vi "get_input_configuration.vi"(8 "error in (no error)":errorcluster, 11 "connection ID":refnum<k5>) -> (0 "error out":errorcluster, 1 "Sensor info 1":T1="1", 2 "Sensor type":T2="0", 3 "connection ID out":refnum<k5>, 4 "Sensor info 2":string)   [LabVIEW 2018]
uses:
  typedefs/sensor_types.ctl
  typedefs/thermocouple_types.ctl
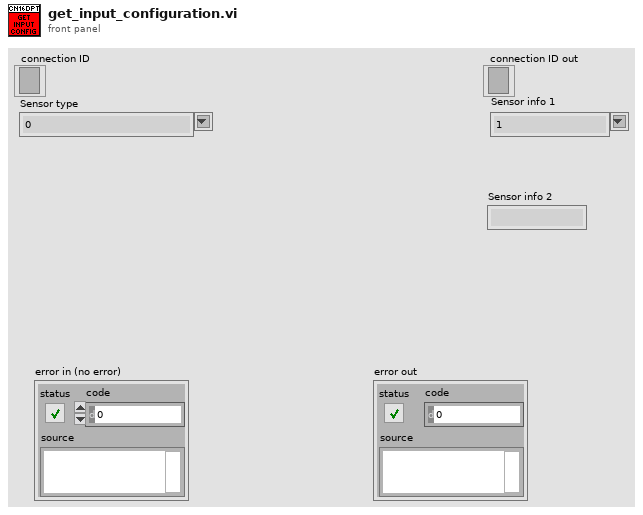
[diagram p1: front panel]
types:
  T1 = typedef "thermocouple_types.ctl" = string
  T2 = typedef "sensor_types.ctl" = string
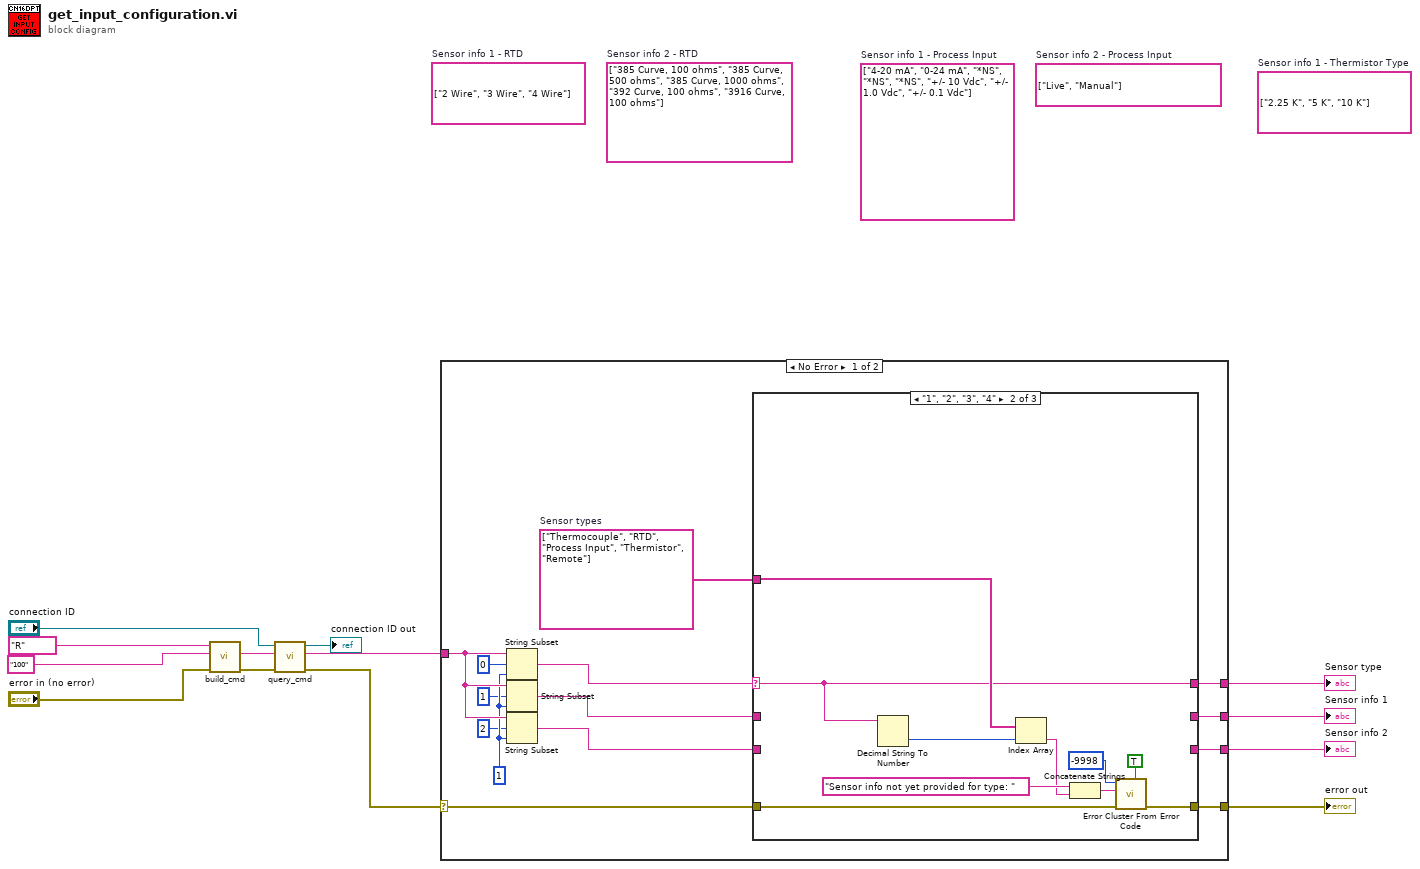
[diagram p0: block diagram]
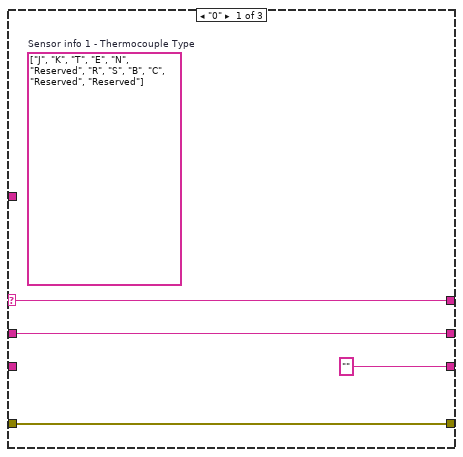
[diagram p2: hidden frame]
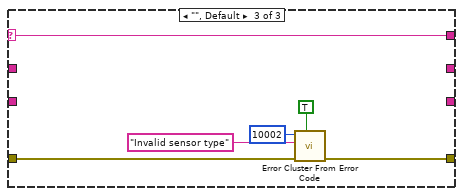
[diagram p3: hidden frame]
diagram:
  (unwired) string[] ["2.25 K", "5 K", "10 K"]  # Sensor info 1 - Thermistor Type
  (unwired) string[] ["Live", "Manual"]  # Sensor info 2 - Process Input
  (unwired) string[] ["4-20 mA", "0-24 mA", "*NS", "*NS", "*NS", "+/- 10 Vdc", "+/- 1.0 Vdc", "+/- 0.1 Vdc"]  # Sensor info 1 - Process Input
  (unwired) string[] ["385 Curve, 100 ohms", "385 Curve, 500 ohms", "385 Curve, 1000 ohms", "392 Curve, 100 ohms", "3916 Curve, 100 ohms"]  # Sensor info 2 - RTD
  (unwired) string[] ["2 Wire", "3 Wire", "4 Wire"]  # Sensor info 1 - RTD
  n1 = call "build_cmd.vi"("error in (no error)"="error in (no error)", "Command ID"="100", "Command class"="R") -> ("error out"=w9:errorcluster, "Command"=w8:string)  [unwired: 7 in]
  n2 = call "query_cmd.vi"("error in (no error)"=w9, "Command"=w8, "connection ID"="connection ID") -> ("error out"=w6:errorcluster, "Response"=w7:string, "connection ID out"=→"connection ID out":refnum<k5>)  [unwired: 6 in]
  n3 = case shown="No Error" w6 {
    selector: w6 -> [w19 w48]
    tunnel: w7 -> [w27 _]
    tunnel: [w22 _] -> w2
    tunnel: [w21 _] -> w1
    tunnel: [w20 _] -> w5
    tunnel: [w18 w48] -> w3
    frame No Error {
      w14 = string[] ["Thermocouple", "RTD", "Process Input", "Thermistor", "Remote"]  # Sensor types
      w25 = 1 ("length (rest)")
      n4 = String Subset(string=w27, offset (0)=0, length (rest)=w25) -> (substring=w17:string)
      n5 = String Subset(string=w27, offset (0)=1, length (rest)=w25) -> (substring=w16:string)
      n6 = String Subset(string=w27, offset (0)=2, length (rest)=w25) -> (substring=w15:string)
      n7 = case shown="\"1\", \"2\", \"3\", \"4\"" w17 {
        selector: w17 -> [w31 w38 w47]
        tunnel: [w31 w38 w47] -> w22
        tunnel: [w29 _ _] -> w21
        tunnel: w16 -> [w29 _ _]
        tunnel: ["" _ _] -> w20
        tunnel: w19 -> [w30 w40 w44]
        tunnel: [w30 w41 w42] -> w18
        tunnel: w15 -> [_ _ _]
        tunnel: w14 -> [_ w39 _]
        frame "0" {
          (unwired) string[] ["J", "K", "T", "E", "N", "Reserved", "R", "S", "B", "C", "Reserved", "Reserved"]  # Sensor info 1 - Thermocouple Type
        }
        frame "1", "2", "3", "4" {
          n8 = Decimal String To Number(string=w38) -> (number=w37:i32)  [unwired: 2 in, 1 out]
          n9 = Index Array(array=w39, index=w37) -> (element=w33:string)
          n10 = Concatenate Strings("Sensor info not yet provided for type: " ("error message (\"\")"), w33) -> (w35:string)
          n11 = call <vilib>:"Error Cluster From Error Code.vi"("is warning? (False)"=TRUE, "error in (no error)"=w40, "error message (\"\")"=w35, "error code (0)"=-9998) -> ("error out"=w41:errorcluster)  [unwired: 5 in]
        }
        frame "", Default {
          n12 = call <vilib>:"Error Cluster From Error Code.vi"("show call chain? (False)"=TRUE, "error in (no error)"=w44, "error message (\"\")"="Invalid sensor type" ("error message (\"\")"), "error code (0)"=10002) -> ("error out"=w42:errorcluster)  [unwired: 5 in]
        }
      }
    }
    frame Error {
    }
  }
  "error out" <- w3
  "Sensor info 2" <- w5
  "Sensor type" <- w2
  "Sensor info 1" <- w1
